vi "CRYProject Editor PIC Get Update State.vi"() -> (0 "bNewState":bool, 2 "bChangeState":bool)   [LabVIEW 2013]
uses:
  CRYProject Editor Global.vi
  CRYMainGlobal.vi
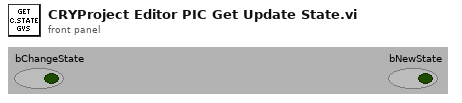
[diagram p1: front panel]
types:
  T1 = typedef "CRYTS.ctl" = cluster{"No.TS":u16, "TS File Path":path, "TS Name":string, "EditStepName":string, "Steps":T2[], "New State":bool, "Change State":bool, "Flattened CurveLib Data":string, "Document Data":string, "EditStepNo":u16, "Operator Start File":string, "Sequence Type":string, "Sequence Language":string}
  T2 = typedef "CRYStep.ctl" = cluster{"No.VI":i32, "Category":string, "StepName":string, "Seq setup flattened":string, "Comment":string, "Steps config.":bool[], "Jump config":i32[], "Start":dbl, "Increment":dbl, "Name":string, "Unit":string, "Y data":u16, "Y prefix":string, "Y dB ref":dbl, "Y unit":string, "Repeat State Array":cluster{"Start":dbl, "Increment":dbl, "Count":i32, "Num":i32}[]}
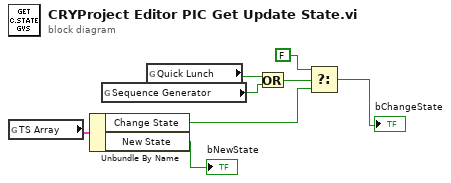
[diagram p0: block diagram]
diagram:
  n1 = global read "CRYProject Editor Global.vi" "TS Array"() -> (w8:T1)
  n2 = Unbundle By Name(w8) -> ("Change State"=w2:bool, "New State"=→"bNewState":bool)
  n3 = global read "CRYMainGlobal.vi" "Sequence Generator"() -> (w5:bool)
  n4 = global read "CRYMainGlobal.vi" "Quick Lunch"() -> (w6:bool)
  n5 = Or(x=w6, y=w5) -> (x .or. y?=w4:bool)
  n6 = Select(t=FALSE, s=w4, f=w2) -> (s? t:f=→"bChangeState":bool)
